vi "Stop Total.vi"(8 "error in (no error)":errorcluster, 11 "User Interface in":refnum<class "User Interface.lvclass">) -> (0 "error out":errorcluster, 3 "User Interface out":refnum<class "User Interface.lvclass">)   [LabVIEW 2020, in "User Interface.lvlib" / "User Interface.lvclass"]
uses:
  User Interface.lvclass
  User Interface.lvclass/User Interface.ctl
  <vilib>/ActorFramework/Message Enqueuer/Message Enqueuer.lvclass/Message Enqueuer.ctl
  <vilib>/ActorFramework/Message Enqueuer/Enqueue.vi
  Manejo Turnos Messages/Stop Total Turnos Msg/Stop Total Turnos Msg.lvclass
  C:/Program Files (x86)/National Instruments/LabVIEW 2020/vi.lib/ActorFramework/Message/Message.lvclass
  <vilib>/ActorFramework/Message Priority Queue/Priority Enqueue.vi
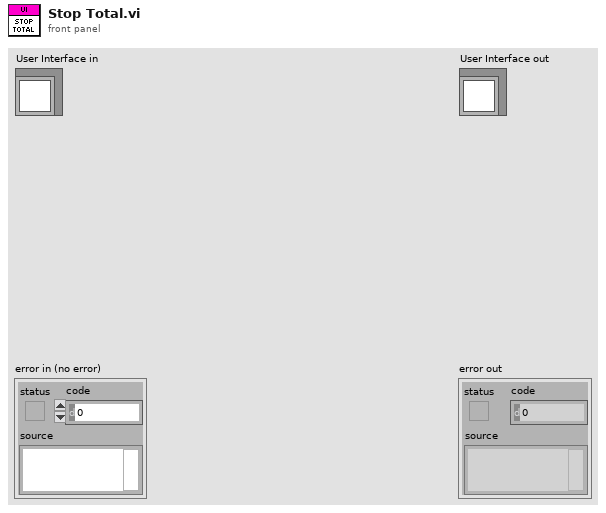
[diagram p1: front panel]
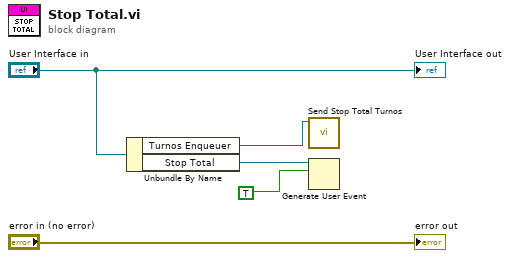
[diagram p0: block diagram]
diagram:
  n1 = Unbundle By Name("User Interface in") -> ("Turnos Enqueuer"=w1:refnum<class "Message Enqueuer.lvclass">, "Stop Total"=w3:refnum<user-event>)
  n2 = call "Send Stop Total Turnos.vi"("Message Enqueuer"=w1) -> ()  [unwired: 9 in, 2 out]
  n3 = Generate User Event(user event=w3, event data cluster=TRUE) -> ()  [unwired: 2 in, 2 out]
  "error out" <- "error in (no error)"
  "User Interface out" <- "User Interface in"
